vi "InitAnalysis.vi"(8 "error in (no error)":errorcluster, 10 "ModuleID":i32, 11 "AnalysisPluginsBase in":refnum<class "AnalysisPluginsBase.lvclass">) -> (0 "error out":errorcluster, 3 "AnalysisPluginsBase out":refnum<class "AnalysisPluginsBase.lvclass">)   [LabVIEW 2018, in "AnalysisPlugins.lvlib" / "AnalysisPluginsBase.lvclass"]
uses:
  AnalysisPluginsBase.lvclass
  Typedefs/clSensorData.ctl
  AnalysisPluginsBase.lvclass/AnalysisPluginsBase.ctl
  Accessors/Write SensorQue.vi
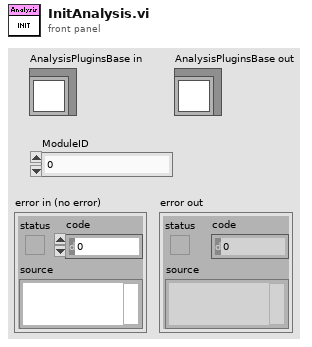
[diagram p1: front panel]
types:
  T1 = typedef "AnalysisPlugins.lvlib/AnalysisPluginsBase.lvclass/clSensorData.ctl" = cluster{"SensorType":string, "SensorData":variant}
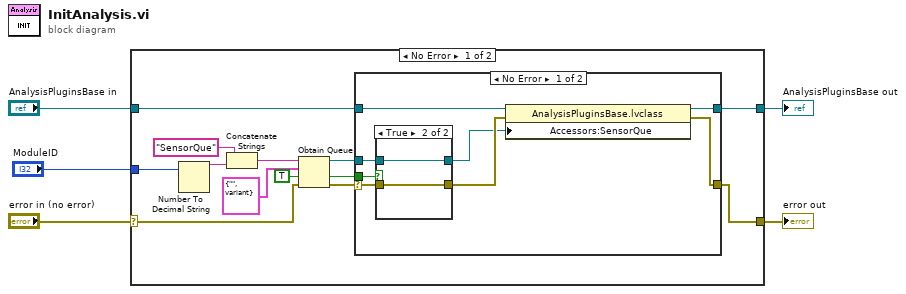
[diagram p0: block diagram]
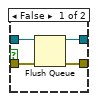
[diagram p2: hidden frame]
diagram:
  n1 = case shown="No Error" "error in (no error)" {
    selector: "error in (no error)" -> [w13 w36]
    tunnel: [w7 w36] -> w4
    tunnel: [w6 w35] -> w2
    tunnel: "AnalysisPluginsBase in" -> [w11 w35]
    tunnel: "ModuleID" -> [w12 _]
    frame No Error {
      n2 = Number To Decimal String(number=w12) -> (decimal integer string=w14:string)  [unwired: 1 in]
      n3 = Concatenate Strings("SensorQue" ("name (unnamed)"), w14) -> (w16:string)
      n4 = Obtain Queue(name (unnamed)=w16, element data type=T1 {"SensorType"="", "SensorData"=variant} ("clSensorData"), create if not found? (T)=TRUE, error in (no error)=w13) -> (queue out=w8:refnum<queue>, created new?=w9:bool, error out=w10:errorcluster)  [unwired: 1 in]
      n5 = case shown="No Error" w10 {
        selector: w10 -> [w25 w34]
        tunnel: w11 -> [w26 w33]
        tunnel: [w19 w34] -> w7
        tunnel: w9 -> [w23 _]
        tunnel: w8 -> [w24 _]
        tunnel: [w20 w33] -> w6
        frame No Error {
          n6 = case shown="True" w23 {
            tunnel: w25 -> [w30 w31]
            tunnel: w24 -> [w29 w32]
            tunnel: [w28 w31] -> w22
            tunnel: [w27 w32] -> w21
            frame False {
              n7 = Flush Queue(queue=w29, error in (no error)=w30) -> (queue out=w27:refnum<queue>, error out=w28:errorcluster)  [unwired: 1 out]
            }
            frame True {
            }
          }
          n8 = property class="AnalysisPluginsBase.lvclass"(reference=w26, error in=w22, "Accessors:SensorQue"=w21) -> (reference out=w20:refnum<class "AnalysisPluginsBase.lvclass">, error out=w19:errorcluster)
        }
        frame Error {
        }
      }
    }
    frame Error {
    }
  }
  "error out" <- w4
  "AnalysisPluginsBase out" <- w2
